vi "Setup Power Sensor.vi"(7 "Trigger Source":i32(ring)=3 items=["Bus", "External", "Hold", "Immediate", "Internal A"], 8 "error in (no error)":errorcluster, 9 "Units":u16(ring) items=["dBm", "W"], 10 "Enable Initiate Continuous":bool=TRUE, 11 "VISA Refnum in":refnum<visa-resource-name>) -> (0 "error out":errorcluster, 3 "VISA Refnum out":refnum<visa-resource-name>)   [LabVIEW 2015]
uses:
  <instrlib>/Agilent U2000 Series/Public/Data/Low Level/Initiate (Continuous).vi
  <instrlib>/Agilent U2000 Series/Agilent U2000 Series.lvlib
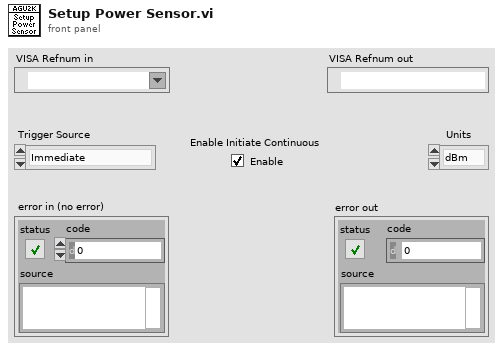
[diagram p1: front panel]
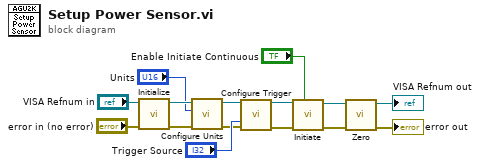
[diagram p0: block diagram]
diagram:
  n1 = call <instrlib>:"Initialize.vi"("error in (no error)"="error in (no error)", "VISA resource name"="VISA Refnum in") -> ("error out"=w10:errorcluster, "VISA resource name out"=w9:refnum<visa-resource-name>)  [unwired: 2 in, 6 out]
  n2 = call <instrlib>:"Configure Units.vi"("error in (no error)"=w10, "Units (0: dBm)"="Units", "VISA resource name"=w9) -> ("error out"=w4:errorcluster, "VISA resource name out"=w3:refnum<visa-resource-name>)  [unwired: 1 in, 6 out]
  n3 = call <instrlib>:"Configure Trigger.vi"("VISA resource name"=w3, "Trigger Source (3: Immediate)"="Trigger Source", "error in (no error)"=w4) -> ("VISA resource name out"=w8:refnum<visa-resource-name>, "error out"=w7:errorcluster)  [unwired: 11 in]
  n4 = call-poly <instrlib>:"Initiate.vi"("Enable Initiate Continuous (T: Enable)"="Enable Initiate Continuous", "error in (no error)"=w7, "VISA resource name"=w8) -> ("error out"=w11:errorcluster, "VISA resource name out"=w12:refnum<visa-resource-name>)  [unwired: 7 in]
  n5 = call <instrlib>:"Zero.vi"("error in (no error)"=w11, "VISA resource name"=w12) -> ("error out"=→"error out":errorcluster, "VISA resource name out"=→"VISA Refnum out":refnum<visa-resource-name>)  [unwired: 8 in]
